vi "balais.vi"() -> ()   [LabVIEW 2019]
uses:
  <vilib>/Rock Robotics/WPI/Solenoid/WPI_SolenoidSetEnum.vi
  <vilib>/Rock Robotics/WPI/Solenoid/WPI_SolenoidValue.ctl
  <vilib>/Rock Robotics/Network Tables/NT Write Boolean.vi
panel:
  in  "bouton\nbouton":bool
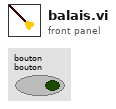
[diagram p1: front panel]
types:
  T1 = typedef "WPI_SolenoidValue.ctl" = enum16{"Off", "On", "Forward", "Reverse"}
  T2 = typedef "WPI_SolenoidDevRef.ctl" = cluster{"DevStatus":errorcluster, "Pneumatics Control Module":u8, "Forward Solenoid Channel":T3, "Reverse Solenoid Channel":T3}
  T3 = typedef "WPI_SolenoidChannel.ctl" = enum8{"Solenoid 0", "Solenoid 1", "Solenoid 2", "Solenoid 3", "Solenoid 4", "Solenoid 5", "Solenoid 6", "Solenoid 7", "Invalid"}
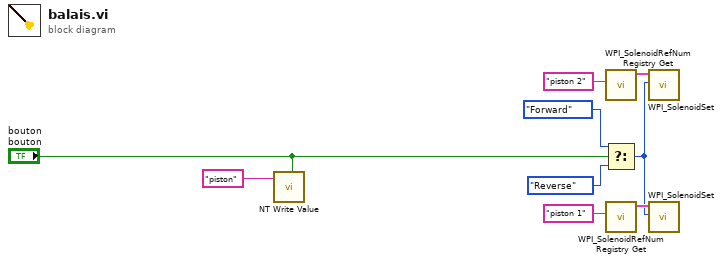
[diagram p0: block diagram]
diagram:
  n1 = call-poly <vilib>:"NT Write Value.vi"("Boolean"="bouton\nbouton", "Name"="piston") -> ()  [unwired: 9 in, 1 out]
  n2 = call <vilib>:"WPI_SolenoidRefNum Registry Get.vi"("refnum name"="piston 2") -> ("SolenoidDevRef"=w6:T2)  [unwired: 9 in, 1 out]
  n3 = Select(t=WPI_SolenoidValue."Forward" ("Value"), s="bouton\nbouton", f=WPI_SolenoidValue."Reverse" ("Value")) -> (s? t:f=w3:T1)
  n4 = call <vilib>:"WPI_SolenoidRefNum Registry Get.vi"("refnum name"="piston 1") -> ("SolenoidDevRef"=w5:T2)  [unwired: 9 in, 1 out]
  n5 = call-poly <vilib>:"WPI_SolenoidSet.vi"("Value"=w3, "SolenoidDevRef"=w6) -> ()  [unwired: 8 in, 2 out]
  n6 = call-poly <vilib>:"WPI_SolenoidSet.vi"("Value"=w3, "SolenoidDevRef"=w5) -> ()  [unwired: 8 in, 2 out]
